vi "MyReadMagField.vi"(8 "error in (no error)":errorcluster, 11 "VISA resource name in":refnum<visa-resource-name>="TCPIP0::192.168.0.107::33576::SOCKET") -> (0 "error out":errorcluster, 1 "B":dbl, 3 "VISA resource name out":refnum<visa-resource-name>)   [LabVIEW 2025, in "MyTriton.lvlib"]
uses:
  MyTriton.lvlib
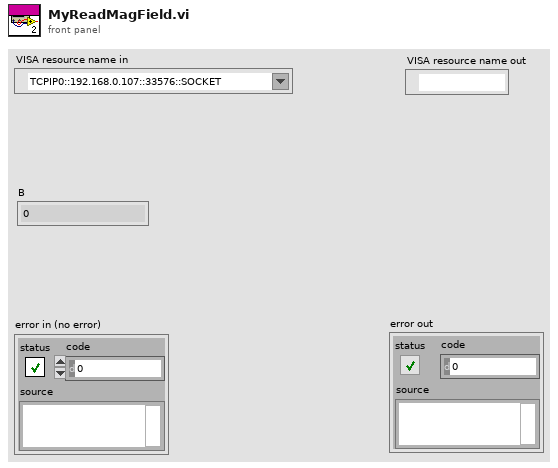
[diagram p1: front panel]
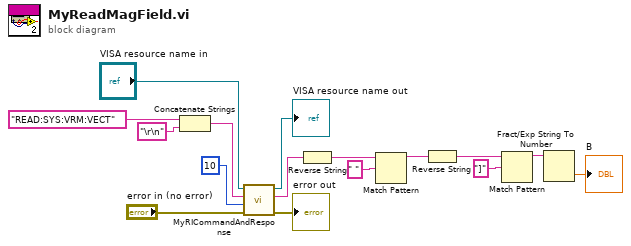
[diagram p0: block diagram]
diagram:
  n1 = Concatenate Strings("READ:SYS:VRM:VECT" ("Command"), "\r\n" ("string")) -> (w14:string)
  n2 = call "MyRICommandAndResponse.vi"("error in (no error)"="error in (no error)", "Min byte count"=u32 10 ("byte count"), "Command"=w14, "VISA resource name in"="VISA resource name in") -> ("error out"=→"error out":errorcluster, "Response"=w5:string, "VISA resource name out"=→"VISA resource name out":refnum<visa-resource-name>)  [unwired: 5 in]
  n3 = Reverse String(1:w5) -> (0:w8:string)
  n4 = Match Pattern(string=w8, regular expression=" ") -> (before substring=w6:string)  [unwired: 1 in, 3 out]
  n5 = Reverse String(1:w6) -> (0:w4:string)
  n6 = Match Pattern(string=w4, regular expression="]") -> (before substring=w2:string)  [unwired: 1 in, 3 out]
  n7 = Fract/Exp String To Number(string=w2) -> (number=→"B":dbl)  [unwired: 3 in, 1 out]
